vi "Make Connection.vi"(6 "Number of Tries":i32=1, 8 "error in (no error)":errorcluster, 11 "IED in":refnum<class "IED.lvclass">) -> (0 "error out":errorcluster, 3 "IED out":refnum<class "IED.lvclass">)   [LabVIEW 2015, in "IED Actor.lvlib" / "IED.lvclass"]
doc: "This VI simply attempts to connect to the Remote Server/IED. A failure at this point should generate error -32190 and should be handled appropriately."
uses:
  IED.lvclass
  IED.lvclass/IED.ctl
  <vilib>/Modbus/master/Create Master Instance (TCP).vi
  <vilib>/Modbus/master/Modbus Master.lvclass
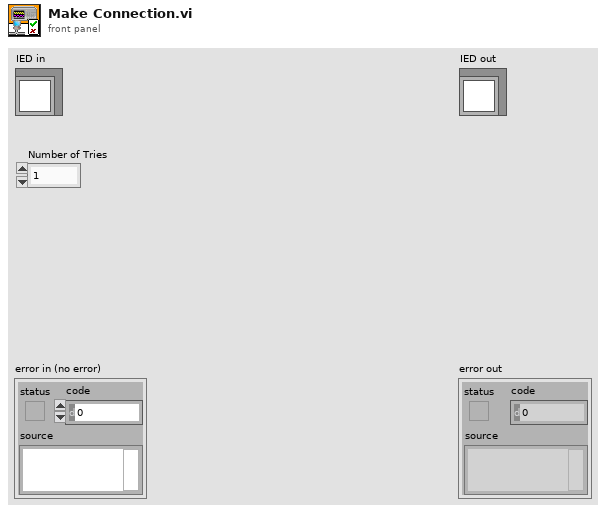
[diagram p1: front panel]
types:
  T1 = typedef "IED Actor.lvlib/IED.lvclass/Comm Cluster.ctl" = cluster{"IP Address":string, "Port":u16}
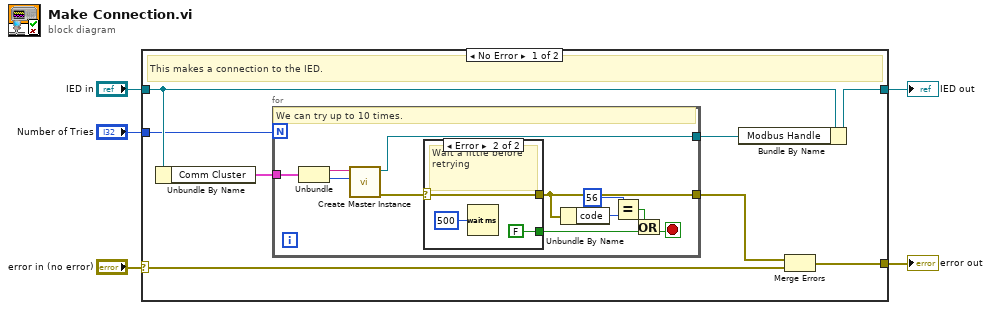
[diagram p0: block diagram]
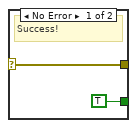
[diagram p2: hidden frame]
diagram:
  n1 = case shown="No Error" "error in (no error)" {
    selector: "error in (no error)" -> [w9 w30]
    tunnel: "IED in" -> [w8 w31]
    tunnel: [w10 w30] -> w4
    tunnel: [w12 w31] -> w3
    tunnel: "Number of Tries" -> [w6 _]
    frame No Error {
      # "This makes a connection to the IED."
      n2 = Unbundle By Name(w8) -> ("Comm Cluster"=w7:T1)
      n3 = for {
        N: w6 -> [_]
        tunnel: w7 -> [w22]
        tunnel: [w21] -> w11
        tunnel: [w17] -> w13
        stop <- w18 stop-if-true
        # "We can try up to 10 times."
        n4 = Unbundle(w22) -> ("IP Address"=w24:string, "Port"=w23:u16)
        n5 = call-poly <vilib>:"Create Master Instance.vi"("port (502)"=w23, "address"=w24) -> ("error out"=w20:errorcluster, "TCP master instance"=w21:refnum<class "Modbus Master.lvclass">)  [unwired: 8 in]
        n6 = case shown="Error" w20 {
          selector: w20 -> [w26 w29]
          tunnel: [w26 w29] -> w17
          tunnel: [TRUE FALSE] -> w19
          frame No Error {
            # "Success!"
          }
          frame Error {
            # "Wait a little before retrying"
            n7 = Wait (ms)(milliseconds to wait=u32 500) -> ()  [unwired: 1 out]
          }
        }
        n8 = Unbundle By Name(w17) -> ("code"=w16:i32)
        n9 = Equal?(x=56, y=w16) -> (x = y?=w14:bool)
        n10 = Or(x=w14, y=w19) -> (x .or. y?=w18:bool)
      }
      n11 = Bundle By Name(cluster=w8, "Modbus Handle"=w11) -> (w12:refnum<class "IED.lvclass">)
      n12 = Merge Errors(w13, w9) -> (w10:errorcluster)
    }
    frame Error {
    }
  }
  "error out" <- w4
  "IED out" <- w3
